vi "Overwrite SensorID.vi"(8 "error in (no error)":errorcluster, 9 "Index":i32, 10 "MSG FetchSensorID Payload":T1, 11 "Instrument Specifications in":T2) -> (0 "error out":errorcluster, 3 "Instrument Specifications out":T2)   [LabVIEW 2026, in "Settings.lvlib"]
uses:
  Settings.lvlib
  Acquisition/Instrument Specifications Configuration.ctl
  Acquisition/Instrument Specifications Cluster Configuration.ctl
  controls/UI/Measurement Role.ctl
  controls/Messaging Payloads/MSG FetchSensorID Payload.ctl
  Acquisition/Acquisition.lvlib
  Database/Database.lvlib
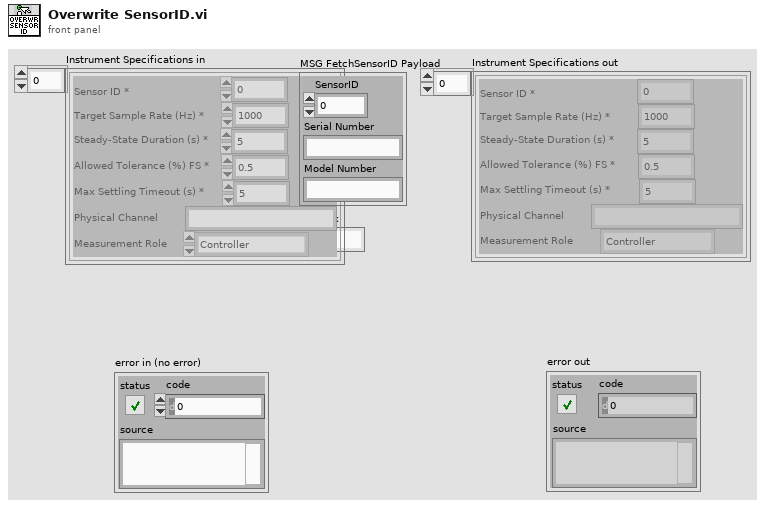
[diagram p1: front panel]
types:
  T1 = typedef "Database.lvlib/MSG FetchSensorID Payload.ctl" = cluster{"SensorID":i32, "Serial Number":string, "Model Number":string}
  T2 = typedef "Acquisition.lvlib/Instrument Specifications Configuration.ctl" = T3[]
  T3 = typedef "Acquisition.lvlib/Instrument Specifications Cluster Configuration.ctl" = cluster{"Sensor ID *":i32, "Target Sample Rate (Hz) *":dbl, "Steady-State Duration (s) *":i32, "Allowed Tolerance (%) FS *":dbl, "Max Settling Timeout (s) *":i32, "Physical Channel":string, "Measurement Role":T4}
  T4 = typedef "Settings.lvlib/Measurement Role.ctl" = enum16{"Controller", "Reference", "UUT", "Disable", "All"}
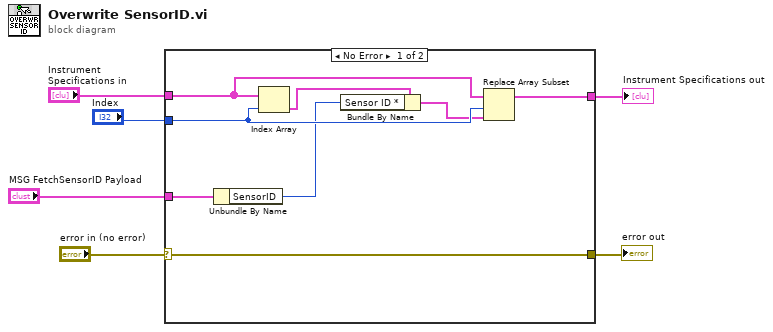
[diagram p0: block diagram]
diagram:
  n1 = case shown="No Error" "error in (no error)" {
    selector: "error in (no error)" -> [w11 w16]
    tunnel: [w14 w15] -> w6
    tunnel: "Index" -> [w13 _]
    tunnel: "Instrument Specifications in" -> [w12 w15]
    tunnel: [w11 w16] -> w2
    tunnel: "MSG FetchSensorID Payload" -> [w8 _]
    frame No Error {
      n2 = Unbundle By Name(w8) -> ("SensorID"=w7:i32)
      n3 = Index Array(array=w12, index=w13) -> (element=w9:T3)
      n4 = Bundle By Name(cluster=w9, "Sensor ID *"=w7) -> (w10:T3)
      n5 = Replace Array Subset(array=w12, new element=w10, index=w13) -> (w14:T2)
    }
    frame Error {
    }
  }
  "Instrument Specifications out" <- w6
  "error out" <- w2
